vi "Write GIF File__ogtk.vi"(7 "overwrite? (false)":bool, 8 "error in (no error)":errorcluster, 10 "image data":T1, 11 "path to GIF file":path) -> (0 "error out":errorcluster, 3 "path":path)   [LabVIEW 2018]
doc: "Writes a single-frame (non-animated) Compuserve GIF file. If no path is specified, a file dialog is used to find the file."
uses:
  <vilib>/picture/picture.llb/imagedata.ctl
panel:
  # "Write GIF File.vi\n\nWrites a single-frame (non-animated) Compuserve GIF file. If no path is specified, a file dialog is used to find the file.\n\nPlease visit http://www.OpenG.org to learn about the\nOpen Source LabVIEW software movement.\n\nNOTICE -- YOU MUST LEAVE THIS NOTICE IN PLACE.  PER THE TERMS OF THE LICENSE BELOW, YOU MAY SUBLICENSE THIS SOFTWARE \nIN ANY WAY THAT DOES NOT CONFLICT WITH THIS LICENSE.\n\n### BSD License (http://www.opensource.org/licenses/bsd-license.php) Begin ###\n \nCopyright (c) 2007, Bill Clench <bclench@yahoo.com>\n\nAll rights reserved.\n\nRedistribution and use in source and binary forms, with or without modification, are permitted provided that the following conditions are met:\n\n    * Redistributions of source code must retain the above copyright notice, this list of conditions and the following disclaimer.\n    * Redistributions in binary form must reproduce the above copyright notice, this list of conditions and the following disclaimer in the \n       documentation and/or other materials provided with the distribution.\n    * Neither the name of SciWare, James Kring, Inc., nor the names of its contributors may be used to endorse or promote products derived \n       from this software without specific prior written permission.\n\nTHIS SOFTWARE IS PROVIDED BY THE COPYRIGHT HOLDERS AND CONTRIBUTORS \"AS IS\" AND ANY EXPRESS OR IMPLIED WARRANTIES, \nINCLUDING, BUT NOT LIMITED TO, THE IMPLIED WARRANTIES OF MERCHANTABILITY AND FITNESS FOR A PARTICULAR PURPOSE ARE \nDISCLAIMED. IN NO EVENT SHALL THE COPYRIGHT OWNER OR CONTRIBUTORS BE LIABLE FOR ANY DIRECT, INDIRECT, INCIDENTAL,\n SPECIAL, EXEMPLARY, OR CONSEQUENTIAL DAMAGES (INCLUDING, BUT NOT LIMITED TO, PROCUREMENT OF SUBSTITUTE GOODS OR \nSERVICES; LOSS OF USE, DATA, OR PROFITS; OR BUSINESS INTERRUPTION) HOWEVER CAUSED AND ON ANY THEORY OF LIABILITY, \nWHETHER IN CONTRACT, STRICT LIABILITY, OR TORT (INCLUDING NEGLIGENCE OR OTHERWISE) ARISING IN ANY WAY OUT OF THE USE \nOF THIS SOFTWARE, EVEN IF ADVISED OF THE POSSIBILITY OF SUCH DAMAGE.\n\n### BSD License End ###"
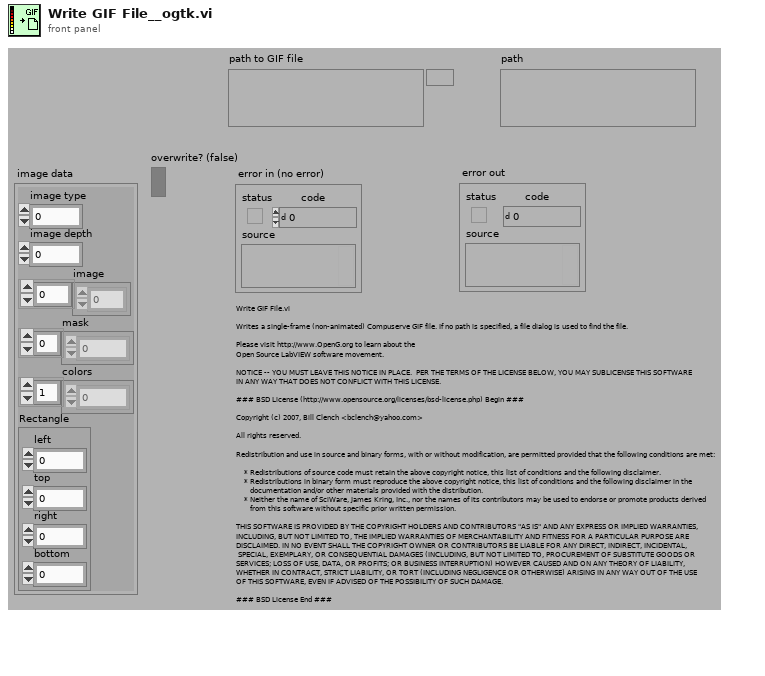
[diagram p1: front panel]
types:
  T1 = typedef "imagedata.ctl" = cluster{"image type":i32, "image depth":i32, "image":u8[], "mask":u8[], "colors":u32[], "Rectangle":cluster{"left":i16, "top":i16, "right":i16, "bottom":i16}}
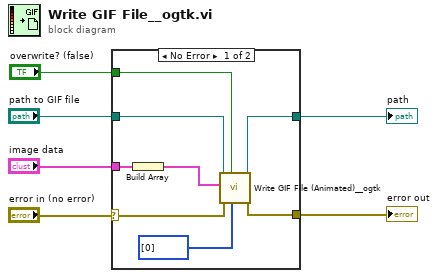
[diagram p0: block diagram]
diagram:
  n1 = case shown="No Error" "error in (no error)" {
    selector: "error in (no error)" -> [w7 w15]
    tunnel: "image data" -> [w14 _]
    tunnel: [w13 w15] -> w5
    tunnel: "path to GIF file" -> [w12 w16]
    tunnel: [w10 w16] -> w3
    tunnel: "overwrite? (false)" -> [w9 _]
    frame No Error {
      n2 = Build Array(w14) -> (w8:T1[])
      n3 = call <userlib>:"Write GIF File (Animated)__ogtk.vi"("delay (ms)"=u16[] [0], "overwrite? (false)"=w9, "error in (no error)"=w7, "images data"=w8, "path to GIF file"=w12) -> ("error out"=w13:errorcluster, "path"=w10:path)  [unwired: 5 in]
    }
    frame Error {
    }
  }
  "error out" <- w5
  "path" <- w3
